vi "Actor Core.vi"(8 "error in":errorcluster, 11 "HIJ JETI100 F and E Camera In":refnum<class "HIJ Vision App Fluence @ fix Energy Camera.lvclass">) -> (0 "error out":errorcluster, 3 "Actor out":refnum<class "Actor.lvclass">)   [LabVIEW 2014, in "HIJ Vision App Fluence @ fix Energy Camera.lvlib" / "HIJ Vision App Fluence @ fix Energy Camera.lvclass"]
doc: "(<B>Filename</B>: Actor Framework.lvlib:Actor.lvclass:Actor Core.vi)\n\nReceives messages to the actor, reacts to them, and initiates any error handling that may shut the actor down.\n\nDescendant classes may override this VI to append parallel tasks for the actor to complete while it handles messages. Overrides use the Call Parent Method node."
uses:
  HIJ Vision App Fluence @ fix Energy Camera.lvclass
  <vilib>/ActorFramework/Actor/Actor.lvclass
  Display Actors/HIJ IMAQdx Display/AF IMAQ Display/HIJ IMAQdx Display.lvclass
  Analyze/Analyze Classes/Analyze Diviation/Analyze BeamDeviation.lvclass
  Analyze/Results and Overlays/Results Beam Deviation/Analyze Results Beam Deviation.lvclass
  Camera Actors/IMAQdx Actor/IMAQdx Actor/IMAQdx Actor.lvclass
  Analyze/Results and Overlays/Results Fluence/Analyze Results Fluence.lvclass
  Analyze/Analyze Parameter/Analyze Parameter Fluence/Analyze Parameter Fluence.lvclass
  Analyze/Analyze Classes/Analyze Fluence/Analyze Fluence.lvclass
  Analyze/Analyze Parameter/Analyze Parameter Energy/Analyze Parameter Energy.lvclass
  Analyze/Analyze Parameter/Analyze Parameter Energy/Analyze Parameter Energy.lvclass/Analyze Parameter Energy.ctl
  Display Actors/HIJ Vision Display/HIJ Vision Display/HIJ Vision Display.lvclass/HIJ Vision Display.ctl
  HIJ Vision App Fluence @ fix Energy Camera.lvclass/HIJ Vision App Fluence @ fix Energy Camera.ctl
  Analyze/Results and Overlays/Results Fluence/Analyze Results Fluence.lvclass/Analyze Results Fluence.ctl
  Applications/HIJ Vision Application/HIJ Vision Application/HIJ Vision Application.lvclass/HIJ Vision Application.ctl
  Applications/HIJ Vision Camera App/HIJ Vision Camera App/HIJ Vision Camera App.lvclass/HIJ Vision Camera App.ctl
  Shared Code/Viewable Actor/ViewableActor/ViewableActor.lvclass/ViewableActor.ctl
  <vilib>/ActorFramework/Actor/Actor.lvclass/Actor.ctl
  <vilib>/ActorFramework/Message Enqueuer/Message Enqueuer.lvclass/Message Enqueuer.ctl
  Applications/HIJ Vision Camera App/HIJ Vision Camera App Messages/Menu Selection Msg/Menu Selection Msg.lvclass/Menu Selection Msg.ctl
  Analyze/Analyze Parameter/Analyze Parameter Energy/Write Energy.vi
  Display Actors/HIJ Vision Display/HIJ Vision Display/Write Save Report_.vi
  Analyze/Results and Overlays/Results Fluence/Write UI Ref Max F.vi
  Applications/HIJ Vision Application/HIJ Vision Application/Write SubPnl for Display.vi
  Applications/HIJ Vision Camera App/HIJ Vision Camera App/Write Child Menu.vi
  Applications/HIJ Vision Application/HIJ Vision Application/Write HIJ Vision Display.vi
  Applications/HIJ Vision Camera App/HIJ Vision Camera App/Write Camera Actor.vi
  Shared Code/Viewable Actor/ViewableActor/Write UI VI Ref.vi
  Applications/HIJ Vision Application/HIJ Vision Application/Write Analyze Objs.vi
  <vilib>/ActorFramework/Message Enqueuer/Init from Existing Queue.vi
  <vilib>/ActorFramework/Message Enqueuer/Enqueue.vi
  <vilib>/ActorFramework/Message Priority Queue/Priority Enqueue.vi
  <vilib>/ActorFramework/Message Enqueuer/Message Enqueuer.lvclass
  Applications/HIJ Vision Camera App/HIJ Vision Camera App Messages/Menu Selection Msg/Menu Selection Msg.lvclass
  <vilib>/ActorFramework/Stop Msg/Stop Msg.lvclass
  Applications/HIJ Vision Camera App/HIJ Vision Camera App/HIJ Vision Camera App.lvclass
panel:
  in  "Stop Button":bool
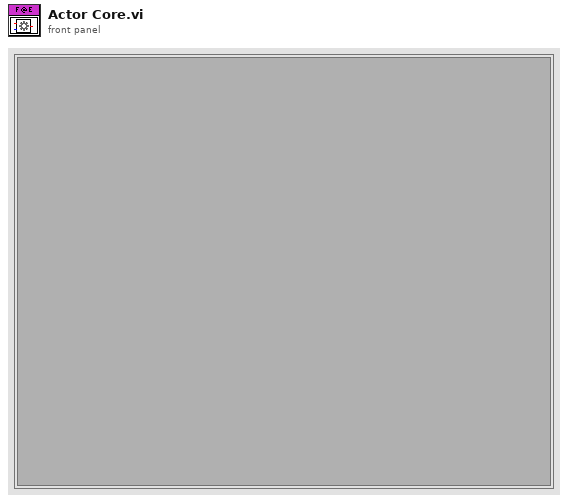
[diagram p1: front panel]
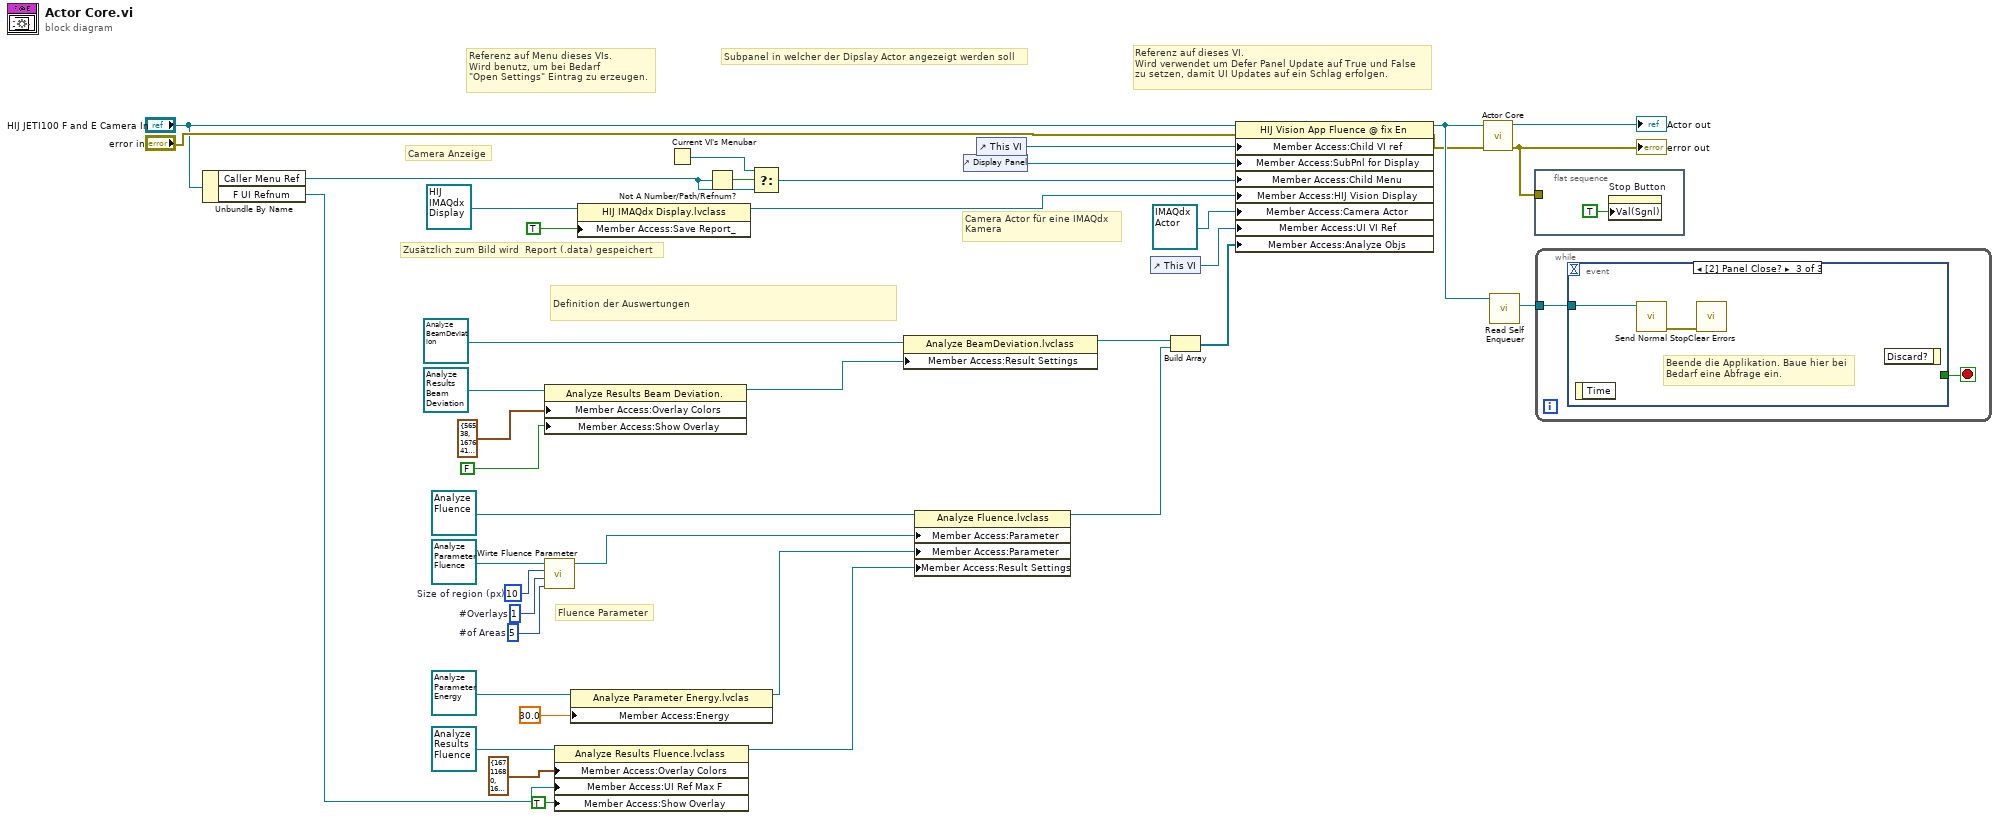
[diagram p0: block diagram]
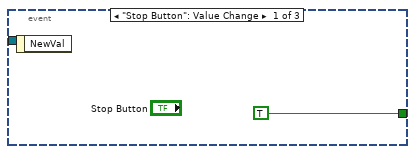
[diagram p2: hidden frame]
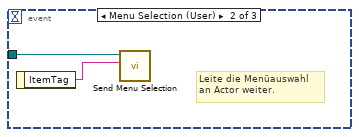
[diagram p3: hidden frame]
diagram:
  w19 = 10  # Size of region (px)
  w20 = 1  # #Overlays
  w21 = 5  # #of Areas
  # "Camera Actor für eine IMAQdx\nKamera"
  # "Referenz auf Menu dieses VIs.\nWird benutz, um bei Bedarf \n\"Open Settings\" Eintrag zu erzeugen."
  # "Fluence Parameter"
  # "Referenz auf dieses VI.\nWird verwendet um Defer Panel Update auf True und False\nzu setzen, damit UI Updates auf ein Schlag erfolgen."
  # "Definition der Auswertungen"
  # "Camera Anzeige"
  # "Zusätzlich zum Bild wird  Report (.data) gespeichert"
  # "Subpanel in welcher der Dipslay Actor angezeigt werden soll"
  n1 = Unbundle By Name("HIJ JETI100 F and E Camera In") -> ("Caller Menu Ref"=w13:refnum<k9>, "F UI Refnum"=w5:refnum<vi>)
  n2 = property class="Analyze Results Beam Deviation."(reference=refnum<class "Analyze Results Beam Deviation.lvclass"> refnum ("Analyze Results Beam Deviation.lvclass"), "Member Access:Overlay Colors"=cluster{"Border":u32, "Text":u32} {"Border"=56538, "Text"=16764160} ("Colors"), "Member Access:Show Overlay"=FALSE ("Show Overlay")) -> (reference out=w23:refnum<class "Analyze Results Beam Deviation.lvclass">)  [unwired: 1 in, 1 out]
  n3 = call "Wirte Fluence Parameter.vi"("#of Areas"=w21, "#Overlays"=w20, "Size of region (px)"=w19, "Analyze Parameter Fluence in"=refnum<class "Analyze Parameter Fluence.lvclass"> refnum ("Analyze Parameter Fluence.lvclass")) -> ("Analyze Parameter Fluence out"=w7:refnum<class "Analyze Parameter Fluence.lvclass">)  [unwired: 7 in]
  n4 = property class="Analyze Results Fluence.lvclass"(reference=refnum<class "Analyze Results Fluence.lvclass"> refnum ("Analyze Results Fluence.lvclass"), "Member Access:Overlay Colors"=cluster{"Border":u32, "Text":u32} {"Border"=16711680, "Text"=16448250} ("Colors"), "Member Access:UI Ref Max F"=w5, "Member Access:Show Overlay"=TRUE ("Show Overlay")) -> (reference out=w6:refnum<class "Analyze Results Fluence.lvclass">)  [unwired: 1 in, 1 out]
  n5 = property class="Analyze Parameter Energy.lvclas"(reference=refnum<class "Analyze Parameter Energy.lvclass"> refnum ("Analyze Parameter Energy.lvclass"), "Member Access:Energy"=dbl[unit] 30.0 ("Energy")) -> (reference out=w2:refnum<class "Analyze Parameter Energy.lvclass">)  [unwired: 1 in, 1 out]
  n6 = property class="HIJ IMAQdx Display.lvclass"(reference=refnum<class "HIJ IMAQdx Display.lvclass"> refnum ("IMAQ Display.lvlib:IMAQ Display.lvclass"), "Member Access:Save Report_"=TRUE ("Save Report_")) -> (reference out=w26:refnum<class "HIJ IMAQdx Display.lvclass">)  [unwired: 1 in, 1 out]
  n7 = Current VI's Menubar() -> (w14:refnum<k9>)
  n8 = Not A Number/Path/Refnum?(number/path/refnum=w13) -> (NaN/Path/Refnum?=w16:bool)
  n9 = Select(t=w14, s=w16, f=w13) -> (s? t:f=w15:refnum<k9>)
  n10 = property class="Analyze BeamDeviation.lvclass"(reference=refnum<class "Analyze BeamDeviation.lvclass"> refnum ("Analyze.lvlib:Analyze BeamDeviation.lvclass"), "Member Access:Result Settings"=w23) -> (reference out=w24:refnum<class "Analyze BeamDeviation.lvclass">)  [unwired: 1 in, 1 out]
  n11 = property class="Analyze Fluence.lvclass"(reference=refnum<class "Analyze Fluence.lvclass"> refnum ("Analyze.lvlib:Analyze Fluence.lvclass"), "Member Access:Parameter"=w7, "Member Access:Parameter"=w2, "Member Access:Result Settings"=w6) -> (reference out=w8:refnum<class "Analyze Fluence.lvclass">)  [unwired: 1 in, 1 out]
  n12 = control-ref of="Display Panel"() -> (w28:refnum<vi>)
  n13 = control-ref of="This VI"() -> (w31:refnum<vi>)
  n14 = control-ref of="This VI"() -> (w18:refnum<vi>)
  n15 = Build Array(w24, w8) -> (w11:refnum<class "Analyze BaseClass.lvclass">[])
  n16 = property class="HIJ Vision App Fluence @ fix En"(reference="HIJ JETI100 F and E Camera In", error in="error in", "Member Access:Child VI ref"=w31, "Member Access:SubPnl for Display"=w28, "Member Access:Child Menu"=w15, "Member Access:HIJ Vision Display"=w26, "Member Access:Camera Actor"=refnum<class "IMAQdx Actor.lvclass"> refnum ("IMAQdx Actor.lvlib:IMAQdx Actor.lvclass"), "Member Access:UI VI Ref"=w18, "Member Access:Analyze Objs"=w11) -> (reference out=w32:refnum<class "HIJ Vision App Fluence @ fix Energy Camera.lvclass">, error out=w29:errorcluster)
  n17 = call-parent "Actor Core.vi"("error in"=w29, "HIJ Vision Camera App In"=w32) -> ("error out"=w38:errorcluster, "Actor out"=→"Actor out":refnum<class "Actor.lvclass">)  [unwired: 8 in]
  "error out" <- w38
  n18 = call <vilib>:"Read Self Enqueuer.vi"("Actor"=w32) -> ("Self Enqueuer"=w37:refnum<class "Message Enqueuer.lvclass">)  [unwired: 10 in]
  n19 = flat-sequence {
    tunnel: w38 -> [_]
    frame #0 {
      n20 = property on="Stop Button" class="Bool (strict)"("Val(Sgnl)"=TRUE) -> ()  [unwired: 2 in, 2 out]
    }
  }
  n21 = while {
    tunnel: w37 -> [w42]
    stop <- w43 stop-if-true
    n22 = event shown="[2] Panel Close?" {
      selector: _ -> [_ _ _]
      dyn-events: _ -> [_ _ _]
      timeout: _ -> [_ _ _]
      tunnel: [TRUE _ _] -> w43
      tunnel: w42 -> [_ w45 w48]
      event "Stop Button": Value Change {
        n23 = event-data() -> ()  [unwired: 1 in, 1 out]
      }
      event Menu Selection (User) {
        # "Leite die Menüauswahl \nan Actor weiter."
        n24 = event-data() -> ("ItemTag"=w46:string)  [unwired: 1 in]
        n25 = call "Send Menu Selection.vi"("MenuTag"=w46, "Message Enqueuer"=w45) -> ()  [unwired: 8 in, 2 out]
      }
      event Panel Close? {
        # "Beende die Applikation. Baue hier bei\nBedarf eine Abfrage ein."
        n26 = event-data() -> ()  [unwired: 1 in, 1 out]
        n27 = call <vilib>:"Send Normal Stop.vi"("Message Enqueuer"=w48) -> ("error out"=w47:errorcluster)  [unwired: 10 in]
        n28 = call <vilib>:"Clear Errors.vi"("error in (no error)"=w47) -> ()  [unwired: 5 in, 2 out]
        n29 = event-data() -> ()  [unwired: 2 in, 1 out]
      }
    }
  }
